vi "delete_document.vi"(0 "Device In":T2, 11 "error in":errorcluster) -> (4 "Device Out":T1, 6 "Comm":T3, 15 "error out":errorcluster)   [LabVIEW 2019]
uses:
  <userlib>/IoT Devices/_subVIs/HTTPComm.ctl
  _SubVI/Cluster.ctl
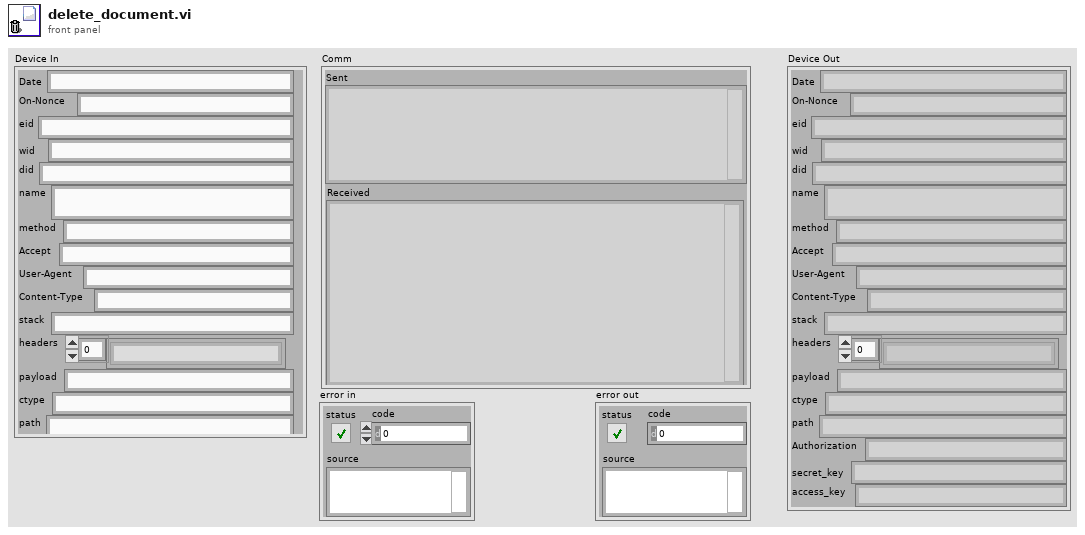
[diagram p1: front panel]
types:
  T1 = typedef "Cluster.ctl" = cluster{"Date":string, "On-Nonce":string, "eid":string, "wid":string, "did":string, "name":string, "method":string, "Accept":string, "User-Agent":string, "Content-Type":string, "stack":string, "headers":string[], "payload":string, "ctype":string, "path":string, "Authorization":string, "secret_key":string, "access_key":string}
  T2 = cluster{"Date":string, "On-Nonce":string, "eid":string, "wid":string, "did":string, "name":string, "method":string, "Accept":string, "User-Agent":string, "Content-Type":string, "stack":string, "headers":string[], "payload":string, "ctype":string, "path":string, "Authorization":string, "secret_key":string, "access_key":string}
  T3 = typedef "HTTPComm.ctl" = cluster{"url":string, "sent headers":string, "sent body":string, "headers":string, "body":string, "Sent":string, "Received":string}
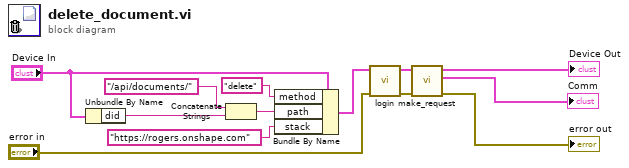
[diagram p0: block diagram]
diagram:
  n1 = Unbundle By Name("Device In") -> ("did"=w4:string)
  n2 = Concatenate Strings("/api/documents/" ("payload"), w4) -> (w11:string)
  n3 = Bundle By Name(cluster="Device In", "method"="delete" ("Method"), "path"=w11, "stack"="https://rogers.onshape.com" ("stacks")) -> (w6:T2)
  n4 = call "login.vi"("error in"="error in", "Device In"=w6) -> ("error out"=w8:errorcluster, "Device Out"=w5:T1)  [unwired: 8 in]
  n5 = call "make_request.vi"("Error in"=w8, "Device In"=w5) -> ("error out"=→"error out":errorcluster, "Comm"=→"Comm":T3, "Device Out"=→"Device Out":T1)  [unwired: 7 in]
